vi "Splitter Test.vi"() -> ()   [LabVIEW 2019]
panel:
  out "Splitter Position":i32
  out "Sizing":T1(ring)
  in  "stop":bool
  in  "Eject Button":bool
  out "Waveform Graph":dbl[](graph)
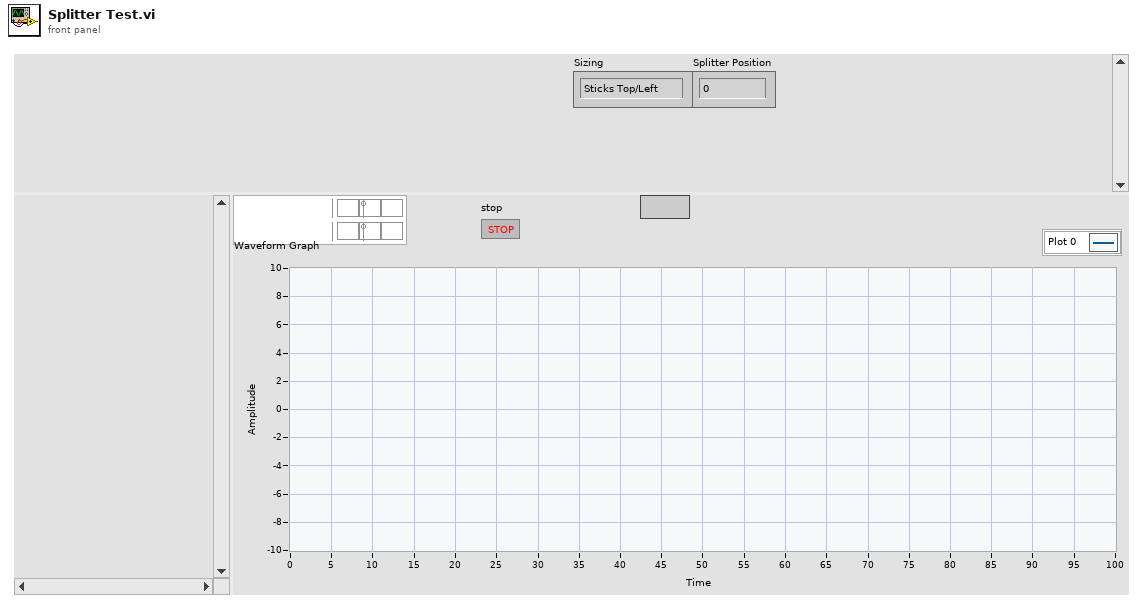
[diagram p1: front panel]
types:
  T1 = enum16{"Sticks Top/Left", "Sticks Bottom/Right", "Proportional"}
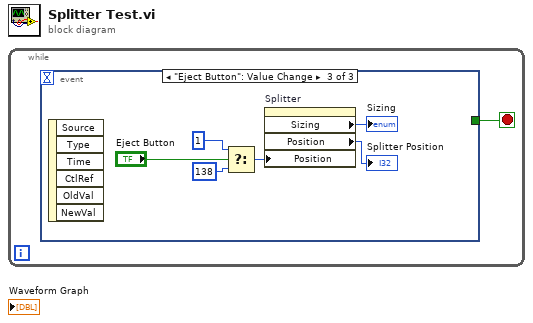
[diagram p0: block diagram]
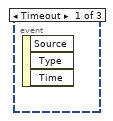
[diagram p2: hidden frame]
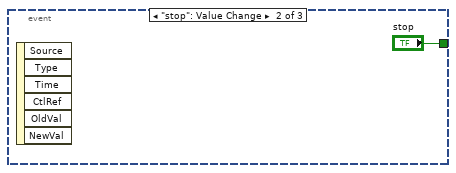
[diagram p3: hidden frame]
diagram:
  n1 = while {
    stop <- w1 stop-if-true
    n2 = event shown="[2] \"Eject Button\": Value Change" {
      selector: _ -> [_ _ _]
      dyn-events: _ -> [_ _ _]
      timeout: _ -> [_ _ _]
      tunnel: [_ "stop" _] -> w1
      event Timeout {
        n3 = event-data() -> ()  [unwired: 1 in, 3 out]
      }
      event "stop": Value Change {
        n4 = event-data() -> ()  [unwired: 1 in, 6 out]
      }
      event "Eject Button": Value Change {
        n5 = event-data() -> ()  [unwired: 1 in, 6 out]
        n6 = Select(t=1 ("Splitter Position"), s="Eject Button", f=138) -> (s? t:f=w3:i32)
        n7 = property on="Splitter" class="Splitter"("Position"=w3) -> ("Sizing"=→"Sizing":T1, "Position"=→"Splitter Position":i32)  [unwired: 2 in, 2 out]
      }
    }
  }
